vi "get_qcm_status.vi"(8 "error in (no error)":errorcluster, 10 "Sensor # (1-indexed)":u8, 11 "VISA resource name":refnum<visa-resource-name>) -> (0 "error out":errorcluster, 2 "QCM status":T1, 3 "VISA resource name out":refnum<visa-resource-name>)   [LabVIEW 2018]
doc: "Query the status of all sensors."
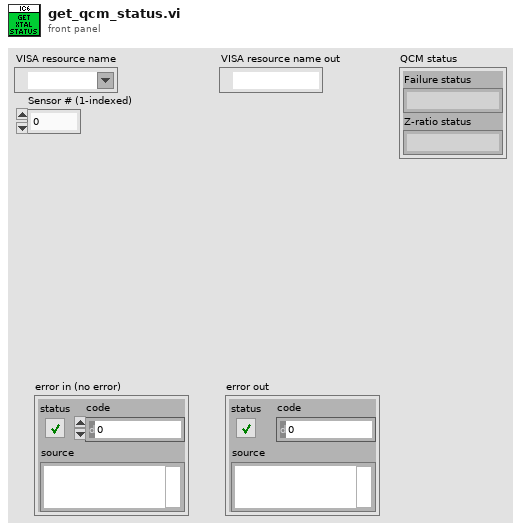
[diagram p1: front panel]
types:
  T1 = cluster{"Failure status":string, "Z-ratio status":string}
  T2 = enum16{"Source", "General", "Input name", "Process name", "Logic", "Material", "Material name", "Output name", "Process", "Sensor", "Output type", "User message", "Layer", ""}
  T3 = enum16{"Hello", "Query", "Remote action", "Status", "Update"}
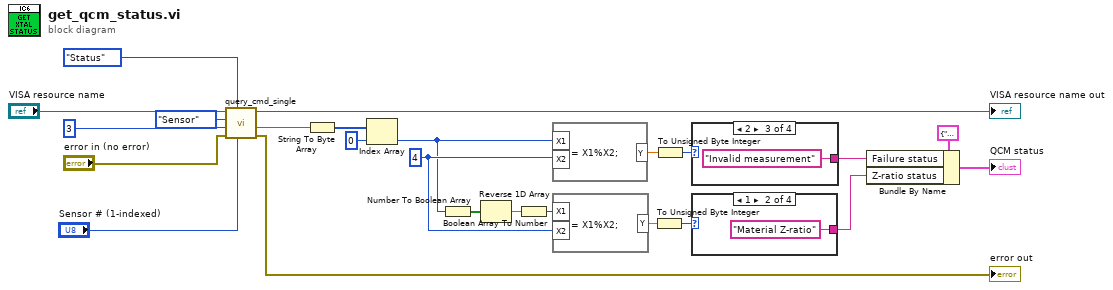
[diagram p0: block diagram]
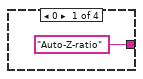
[diagram p2: hidden frame]
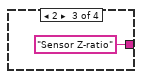
[diagram p3: hidden frame]
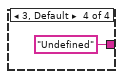
[diagram p4: hidden frame]
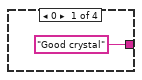
[diagram p5: hidden frame]
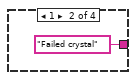
[diagram p6: hidden frame]
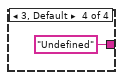
[diagram p7: hidden frame]
diagram:
  w5 = u8 4 ("input variable")
  n1 = call "query_cmd_single.vi"("Parameter"="Sensor # (1-indexed)", "Command group"=T3."Status", "error in (no error)"="error in (no error)", "Command ID"=u8 3, "Command subgroup"=T2."Sensor", "VISA resource name"="VISA resource name") -> ("error out"=→"error out":errorcluster, "formatted response"=w3:string, "VISA resource name out"=→"VISA resource name out":refnum<visa-resource-name>)  [unwired: 1 in, 2 out]
  n2 = String To Byte Array(string=w3) -> (unsigned byte array=w17:u8[])
  n3 = Index Array(array=w17, index=0) -> (element=w4:u8)
  n4 = Number To Boolean Array(number=w4) -> (Boolean array=w13:bool[])
  n5 = Reverse 1D Array(array=w13) -> (reversed array=w12:bool[])
  n6 = Boolean Array To Number(Boolean array=w12) -> (number=w11:u32)
  n7 = formula code="Y = X1%X2;"("X1"=w4, "X2"=w5) -> ("Y"=w9:dbl)
  n8 = formula code="Y = X1%X2;"("X1"=w11, "X2"=w5) -> ("Y"=w10:dbl)
  n9 = To Unsigned Byte Integer(number=w10) -> (unsigned 8bit integer=w7:u8)
  n10 = To Unsigned Byte Integer(number=w9) -> (unsigned 8bit integer=w8:u8)
  n11 = case shown="2" w8 {
    tunnel: ["Good crystal" ("String") "Failed crystal" ("String") "Invalid measurement" ("String") "Undefined" ("String")] -> w14
    frame 0 {
    }
    frame 1 {
    }
    frame 2 {
    }
    frame 3, Default {
    }
  }
  n12 = case shown="1" w7 {
    tunnel: ["Auto-Z-ratio" ("String") "Material Z-ratio" ("String") "Sensor Z-ratio" ("String") "Undefined" ("String")] -> w15
    frame 0 {
    }
    frame 1 {
    }
    frame 2 {
    }
    frame 3, Default {
    }
  }
  n13 = Bundle By Name(cluster=T1 {"Failure status"="", "Z-ratio status"=""}, "Failure status"=w14, "Z-ratio status"=w15) -> (→"QCM status":T1)
